vi "buildTestLog.vi"(8 "error in (no error)":errorcluster, 9 "ScanName":string, 10 "TestLogTypes":T1, 11 "TestLogFactory in":refnum<class "TestLogFactory.lvclass">) -> (0 "error out":errorcluster, 2 "ITestLog":refnum<class "ITestLog.lvclass">, 3 "TestLogFactory out":refnum<class "TestLogFactory.lvclass">)   [LabVIEW 2015, in "TestLogFactory.lvclass"]
uses:
  TestLogFactory.lvclass
  TestLog/ITestLog/ITestLog.lvclass
  Typedefs/TestLogTypes.ctl
  <userlib>/Common/ConfigurationReader/ConfigurationReader.lvclass
  TestLog/CSVTestLog/CSVTestLog.lvclass
  <userlib>/Common/Log/Config/Log.ctl
  View/famtView.vi
  <userlib>/Common/Log/Log.lvlib
  View/FAMTViews.lvlib
  Typedefs/FAMTTypedefs.lvlib
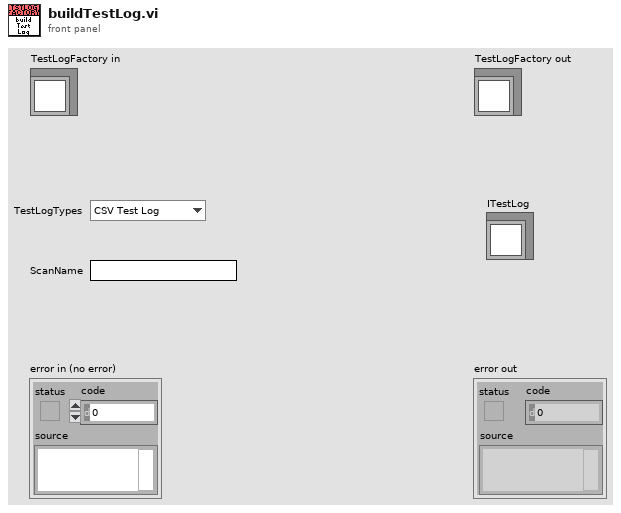
[diagram p1: front panel]
types:
  T1 = typedef "FAMTTypedefs.lvlib/TestLogTypes.ctl" = enum16{"CSV Test Log"}
  T2 = typedef "Log.lvlib/Log.ctl" = cluster{"Log Directory":path, "Log Filename Base":string, "Max records per file":u32, "Comment":string}
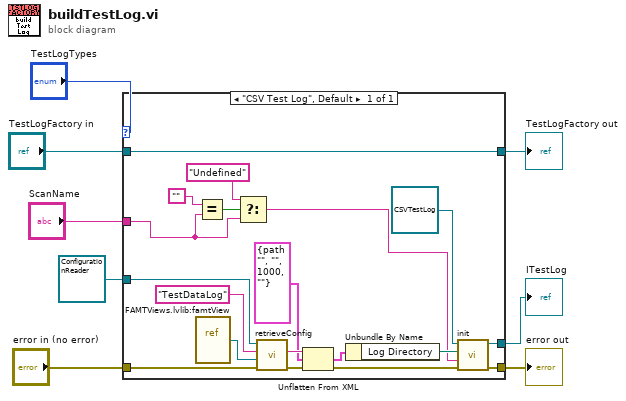
[diagram p0: block diagram]
diagram:
  n1 = case shown="\"CSV Test Log\", Default" "TestLogTypes" {
    tunnel: "error in (no error)" -> [w22]
    tunnel: [w26] -> w2
    tunnel: [w15] -> w3
    tunnel: [w27] -> w1
    tunnel: "TestLogFactory in" -> [w27]
    tunnel: refnum<class "ConfigurationReader.lvclass"> refnum ("ConfigurationReader.lvclass") -> [w24]
    tunnel: "ScanName" -> [w11]
    frame "CSV Test Log", Default {
      n2 = vi-ref "FAMTViews.lvlib:famtView.vi"() -> (w14:refnum<vi>)
      n3 = Equal?(x="", y=w11) -> (x = y?=w12:bool)
      n4 = Select(t="Undefined", s=w12, f=w11) -> (s? t:f=w10:string)
      n5 = call <userlib>:"retrieveConfig.vi"("error in (no error)"=w22, "callingVIRef"=w14, "configName"="TestDataLog", "ConfigurationReader in"=w24) -> ("error out"=w20:errorcluster, "xmlData"=w21:string)  [unwired: 5 in, 1 out]
      n6 = Unflatten From XML(xml string=w21, type=T2 {"Log Directory"=path "", "Log Filename Base"="", "Max records per file"=1000, "Comment"=""} ("Log"), error in (no error)=w20) -> (value=w18:T2, error out=w16:errorcluster)
      n7 = Unbundle By Name(w18) -> ("Log Directory"=w17:path)
      n8 = call "init.vi"("error in (no error)"=w16, "ScanName"=w10, "LogPath"=w17, "CSVTestLog in"=refnum<class "CSVTestLog.lvclass"> refnum ("CSVTestLog.lvclass")) -> ("error out"=w15:errorcluster, "CSVTestLog out"=w26:refnum<class "CSVTestLog.lvclass">)  [unwired: 6 in]
    }
  }
  "error out" <- w3
  "TestLogFactory out" <- w1
  "ITestLog" <- w2
